vi "ReadRSSIInfo.vi"() -> ()   [LabVIEW 2013]
panel:
  out "ReadToEnd":string
  out "Start?":bool
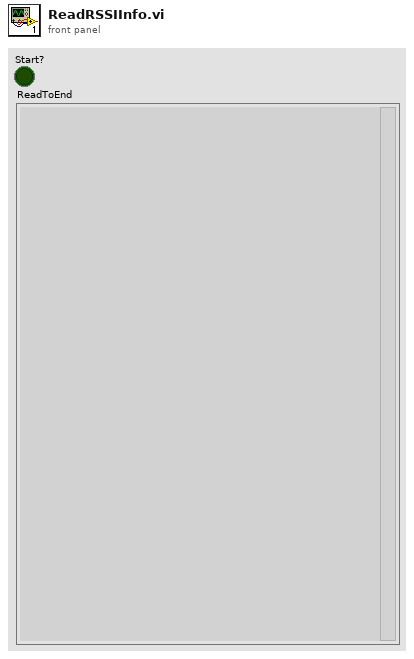
[diagram p1: front panel]
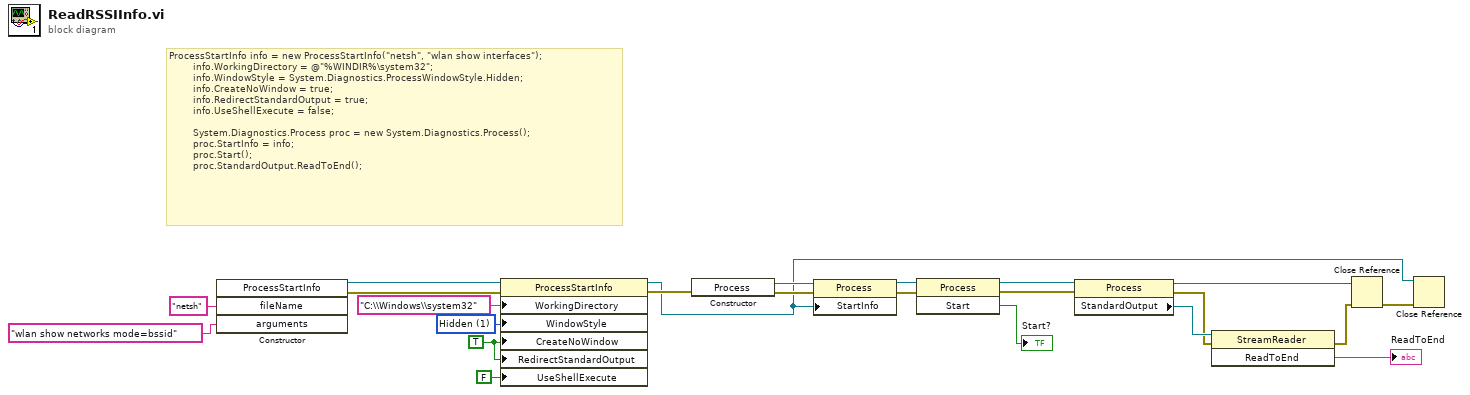
[diagram p0: block diagram]
diagram:
  w17 = TRUE ("CreateNoWindow")
  w18 = 1 items=["Normal", "Hidden", "Minimized", "Maximized"] ("WindowStyle")
  # "ProcessStartInfo info = new ProcessStartInfo(\"netsh\", \"wlan show interfaces\");\n        info.WorkingDirectory = @\"%WINDIR%\\system32\";\n        info.WindowStyle = System.Diagnostics.ProcessWindowStyle.Hidden;\n        info.CreateNoWindow = true;\n        info.RedirectStandardOutput = true;\n        info.UseShellExecute = false;\n\n        System.Diagnostics.Process proc = new System.Diagnostics.Process();\n        proc.StartInfo = info;\n        proc.Start();\n        proc.StandardOutput.ReadToEnd();"
  n1 = constructor class="ProcessStartInfo"("fileName"="netsh", "arguments"="wlan show networks mode=bssid" ("fileName")) -> (reference out=w21:refnum<k24>, error out=w20:errorcluster)  [unwired: 3 in, 3 out]
  n2 = property class="ProcessStartInfo"(reference=w21, error in=w20, "WorkingDirectory"="C:\\Windows\\system32", "WindowStyle"=w18, "CreateNoWindow"=w17, "RedirectStandardOutput"=w17, "UseShellExecute"=FALSE) -> (reference out=w1:refnum<k24>, error out=w13:errorcluster)
  n3 = constructor class="Process"(error in=w13) -> (reference out=w15:refnum<k24>, error out=w14:errorcluster)  [unwired: 2 in, 1 out]
  n4 = property class="Process"(reference=w15, error in=w14, "StartInfo"=w1) -> (reference out=w11:refnum<k24>, error out=w12:errorcluster)
  n5 = invoke class="Process" method="Start"(reference=w11, error in=w12) -> (reference out=w8:refnum<k24>, error out=w7:errorcluster, "Start"=→"Start?":bool)  [unwired: 1 in]
  n6 = property class="Process"(reference=w8, error in=w7) -> (reference out=w3:refnum<k24>, error out=w4:errorcluster, "StandardOutput"=w6:refnum<k24>)
  n7 = invoke class="StreamReader" method="ReadToEnd"(reference=w6, error in=w4) -> (error out=w2:errorcluster, "ReadToEnd"=→"ReadToEnd":string)  [unwired: 1 in, 1 out]
  n8 = Close Reference(reference=w3, error in (no error)=w2) -> (error out=w9:errorcluster)
  n9 = Close Reference(reference=w1, error in (no error)=w9) -> ()  [unwired: 1 out]
